vi "AboutScreen.vi"(11 "Version Info. In":string) -> ()   [LabVIEW 2018]
doc: "*-----------------------------------------------------\n* Author: SWatts\n*\n* VI Description: Displays About dialog\n* \n*\n* Error handling: All errors passed out\n*\n* Pre-condition: \n*\n* Post-condition: None\n*\n* Revision History:\n*\n* Rev Date Author Description \n* 01 30/04/2014 SWatts First issue\n*\n*-----------------------------------------------------"
uses:
  <vilib>/Platform/browser.llb/Open URL in Default Browser (string).vi
panel:
  in  "Website":bool
  in  "Close":bool
  out "Version Info.":string
  out "Version:":string
  # "Copyright 2020, SSDC Ltd"
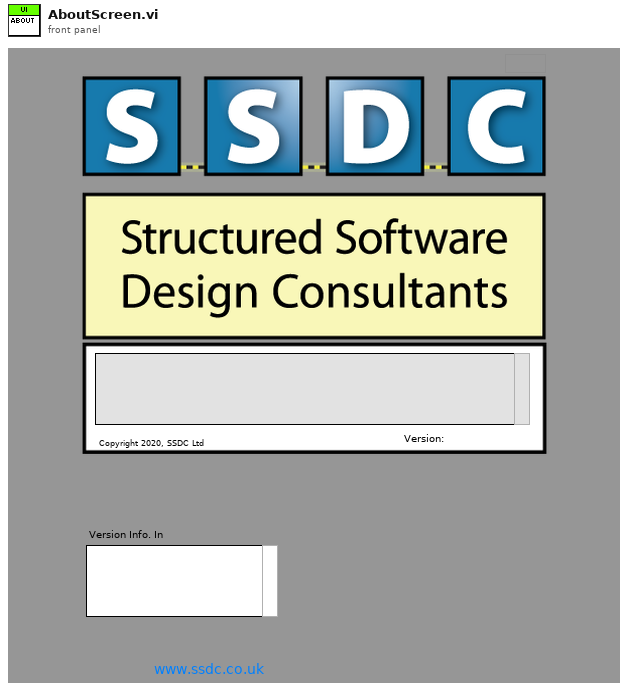
[diagram p1: front panel]
types:
  T1 = enum32{"Invalid", "Standard", "Closed", "Hidden", "Minimized", "Maximized"}
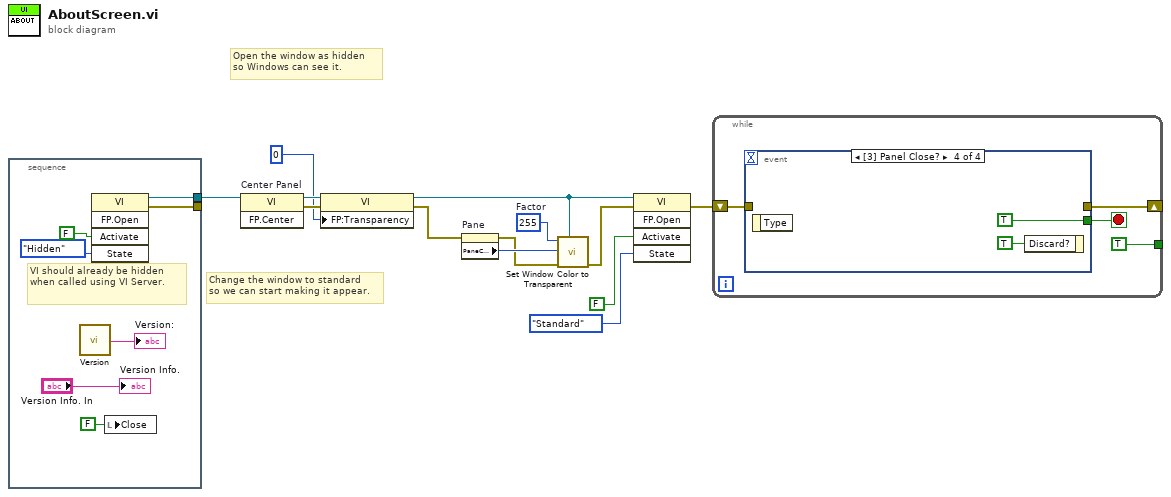
[diagram p0: block diagram]
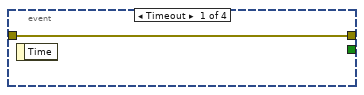
[diagram p2: hidden frame]
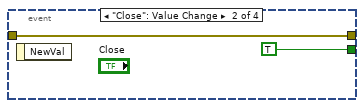
[diagram p3: hidden frame]
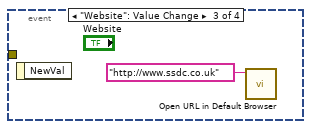
[diagram p4: hidden frame]
diagram:
  w8 = u8 255  # Factor
  # "Change the window to standard\nso we can start making it appear."
  # "Open the window as hidden\nso Windows can see it."
  n1 = stacked-sequence {
    tunnel: [w18] -> w9
    tunnel: [w17] -> _
    frame #0 {
      # "VI should already be hidden when called using VI Server."
      n2 = call "Version.vi"() -> ("Version"=→"Version:":string)  [unwired: 5 in]
      n3 = invoke class="VI" method="FP.Open"("Activate"=FALSE ("Activate?"), "State"=T1."Hidden") -> (reference out=w18:refnum<vi>, error out=w17:errorcluster)  [unwired: 3 in, 3 out]
      n4 = local write "Close"(FALSE ("Close")) -> ()
      "Version Info." <- "Version Info. In"
    }
  }
  n5 = invoke on="Center Panel" class="VI" method="FP.Center"(reference=w9) -> (reference out=w10:refnum<vi>, error out=w11:errorcluster)  [unwired: 2 in, 1 out]
  n6 = property class="VI"(reference=w10, error in=w11, "FP:Transparency"=u8 0 ("t")) -> (reference out=w3:refnum<vi>, error out=w5:errorcluster)
  n7 = property on="Pane" class="Pane"(error in=w5) -> (error out=w6:errorcluster, "PaneColor"=w7:u32)  [unwired: 1 in, 1 out]
  n8 = call "Set Window Color to Transparent.vi"("Calling VI's reference"=w3, "error in (no error)"=w6, "Color to Replace"=w7, "Factor"=w8) -> ("error out"=w4:errorcluster)  [unwired: 4 in]
  n9 = invoke class="VI" method="FP.Open"(reference=w3, error in=w4, "Activate"=FALSE ("Activate?"), "State"=T1."Standard") -> (error out=w1:errorcluster)  [unwired: 1 in, 4 out]
  n10 = while {
    shift-right: [w24] -> _
    shift-left: w1 -> [w21]
    tunnel: [TRUE ("stop")] -> _
    stop <- w23 stop-if-true
    n11 = event shown="[3] Panel Close?" {
      selector: _ -> [_ _ _ _]
      dyn-events: _ -> [_ _ _ _]
      timeout: _ -> [_ _ _ _]
      tunnel: w21 -> [w25 w26 _ _]
      tunnel: [w25 w26 _ _] -> w24
      tunnel: [_ TRUE ("Close") _ TRUE ("Close")] -> w23
      event Timeout {
        n12 = event-data() -> ()  [unwired: 1 in, 1 out]
      }
      event "Close": Value Change {
        n13 = event-data() -> ()  [unwired: 1 in, 1 out]
      }
      event "Website": Value Change {
        n14 = event-data() -> ()  [unwired: 1 in, 1 out]
        n15 = call-poly <vilib>:"Open URL in Default Browser.vi"("URL"="http://www.ssdc.co.uk" ("Link")) -> ()  [unwired: 5 in, 2 out]
      }
      event Panel Close? {
        n16 = event-data() -> ()  [unwired: 1 in, 1 out]
        n17 = event-data("Discard?"=TRUE) -> ()  [unwired: 1 in, 1 out]
      }
    }
  }
